vi "testerrro.vi"() -> ()   [LabVIEW 2011]
panel:
  in  "Up":bool
  in  "Down Button":bool
  in  "stop":bool
  in  "String":string
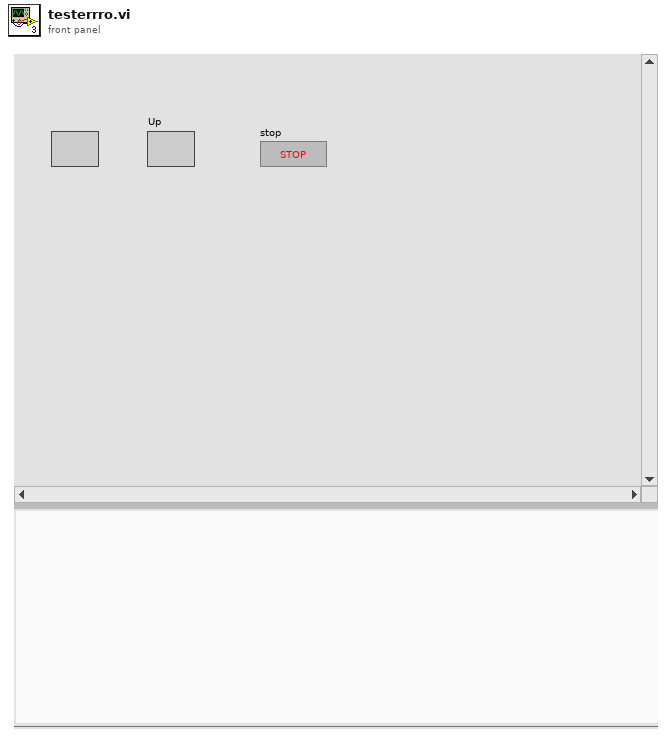
[diagram p1: front panel]
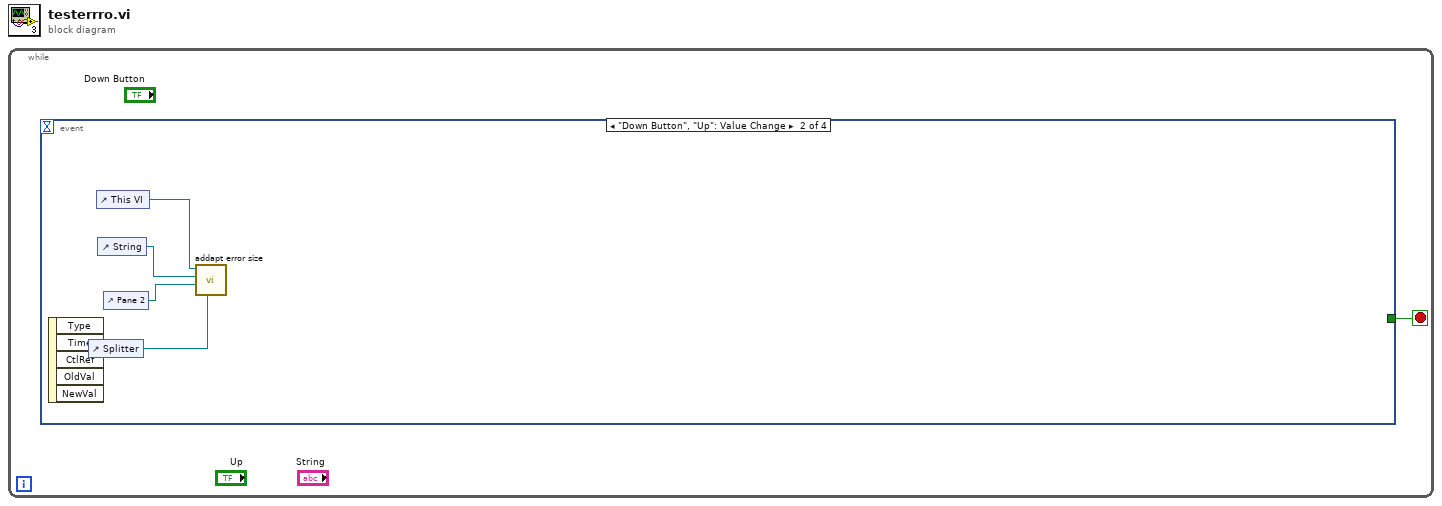
[diagram p0: block diagram]
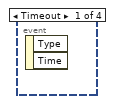
[diagram p2: hidden frame]
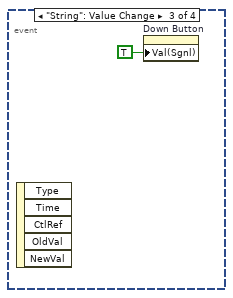
[diagram p3: hidden frame]
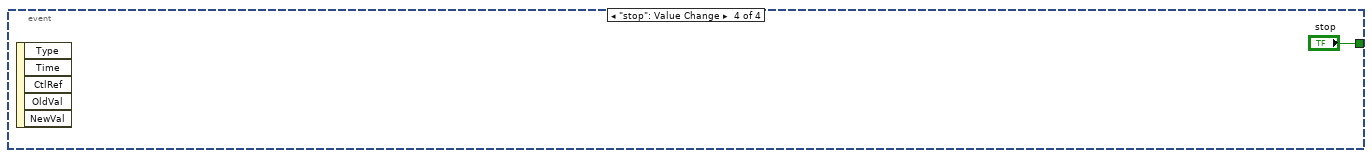
[diagram p4: hidden frame]
diagram:
  n1 = while {
    stop <- w1 stop-if-true
    n2 = event shown="[1] \"Down Button\", \"Up\": Value Change" {
      selector: _ -> [_ _ _ _]
      dyn-events: _ -> [_ _ _ _]
      timeout: _ -> [_ _ _ _]
      tunnel: [_ _ _ "stop"] -> w1
      event Timeout {
        n3 = event-data() -> ()  [unwired: 1 in, 2 out]
      }
      event "Down Button", "Up": Value Change {
        n4 = event-data() -> ()  [unwired: 1 in, 5 out]
        n5 = control-ref of="Splitter"() -> (w5:refnum<vi>)
        n6 = control-ref of="This VI"() -> (w4:refnum<vi>)
        n7 = control-ref of="String"() -> (w3:refnum<vi>)
        n8 = control-ref of="Pane 2"() -> (w2:refnum<vi>)
        n9 = call "addapt error size.vi"("Splitter"=w5, "Pane in"=w2, "String"=w3, "VI in"=w4) -> ()  [unwired: 8 in]
      }
      event "String": Value Change {
        n10 = event-data() -> ()  [unwired: 1 in, 5 out]
        n11 = property on="Down Button" class="Bool (strict)"("Val(Sgnl)"=TRUE) -> ()  [unwired: 2 in, 2 out]
      }
      event "stop": Value Change {
        n12 = event-data() -> ()  [unwired: 1 in, 5 out]
      }
    }
  }
